vi "NumToPercent.vi"(0 "MaxVal":dbl, 1 "MaxOut":u8=255, 2 "MinVal":dbl, 3 "CurVal":dbl, 4 "MinOut":u8) -> (5 "IntPercent":u8)   [LabVIEW 2017, in "ArgosLib.lvlib"]
uses:
  ArgosLib.lvlib
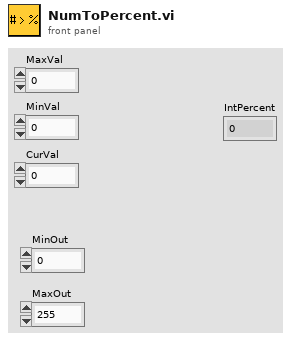
[diagram p1: front panel]
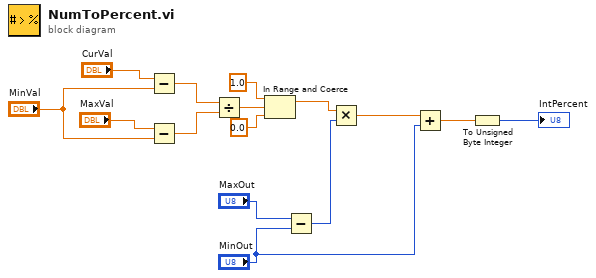
[diagram p0: block diagram]
diagram:
  n1 = Subtract(x="CurVal", y="MinVal") -> (x-y=w14:dbl)
  n2 = Subtract(x="MaxVal", y="MinVal") -> (x-y=w11:dbl)
  n3 = Divide(x=w14, y=w11) -> (x/y=w10:dbl)
  n4 = In Range and Coerce(upper limit=1.0, x=w10, lower limit=0.0) -> (coerced(x)=w7:dbl)  [unwired: 1 out]
  n5 = Subtract(x="MaxOut", y="MinOut") -> (x-y=w4:u8)
  n6 = Multiply(x=w7, y=w4) -> (x*y=w2:dbl)
  n7 = Add(x=w2, y="MinOut") -> (x+y=w1:dbl)
  n8 = To Unsigned Byte Integer(number=w1) -> (unsigned 8bit integer=→"IntPercent":u8)
